vi "Actor Core.vi"(8 "error in":errorcluster, 11 "User Interface":refnum<class "UI.lvclass">) -> (0 "error out":errorcluster, 3 "Actor out":refnum<class "Actor.lvclass">)   [LabVIEW 2017, in "Generic UI Actor.lvlib" / "UI.lvclass"]
doc: "This is Actor Core.vi, the main message handling loop for Actors. An actor usually just sits in this loop and processes messages as they arrive. Any error returned by the message Do.vi call will stop the loop, with error code 43 as the cannonical signal to stop with no error sent to caller. Descendants may override that in Handle Error.vi."
uses:
  UI.lvclass
  <vilib>/ActorFramework/Actor/Actor.lvclass
panel:
  in  "No UI has been defined for this \nmeasurement system":bool
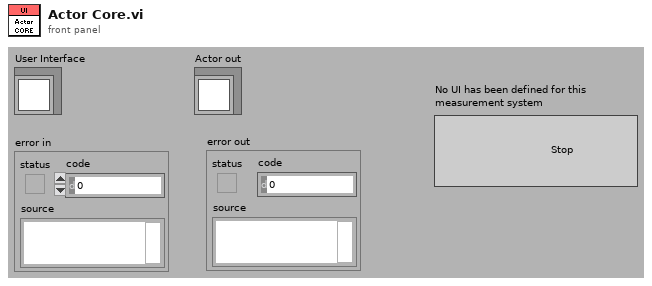
[diagram p1: front panel]
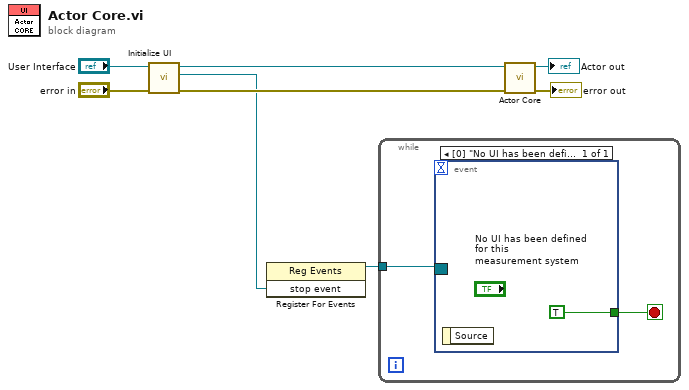
[diagram p0: block diagram]
diagram:
  n1 = call "Initialize UI.vi"("error in (no error)"="error in", "UI in"="User Interface") -> ("error out"=w5:errorcluster, "stop event"=w2:refnum<user-event>, "UI out"=w6:refnum<class "UI.lvclass">)  [unwired: 7 in]
  n2 = register-events(w2) -> (reference out=w1:refnum<event-registration>)  [unwired: 2 in, 1 out]
  n3 = while {
    tunnel: w1 -> [w9]
    stop <- w10 stop-if-true
    n4 = event shown="[0] \"No UI has been defined for this  measurement system\": Value Change;  <stop event>: User Event" {
      selector: w9 -> [_]
      dyn-events: _ -> [_]
      timeout: _ -> [_]
      tunnel: [TRUE] -> w10
      event "No UI has been defined for this \nmeasurement system": Value Change; User Event {
        n5 = event-data() -> ()  [unwired: 1 in, 1 out]
      }
    }
  }
  n6 = call-parent "Actor Core.vi"("error in"=w5, "Actor in"=w6) -> ("error out"=→"error out":errorcluster, "Actor out"=→"Actor out":refnum<class "Actor.lvclass">)  [unwired: 8 in]
